vi "TR_Load_TDMS_for_Repair.vi"(6 "Basic setings cluster":variant, 7 "Decimate?":bool, 8 "error in (no error)":errorcluster, 9 "Post-processing parameters in":variant, 10 "Full settings cluster":variant, 11 "TDMS track":path) -> (0 "error out":errorcluster, 2 "Post-processing parameters out (copy)":variant, 3 "XY data":T1)   [LabVIEW 2018, in "Tracks Repair.lvlib"]
uses:
  Tracks Repair.lvlib
  SubVi's/Controls/CTL_Overlays_cluster.ctl
  SubVi's/Controls/CTL_Full_Track_Array.ctl
  <vilib>/Utility/miscctls.llb/LVBoundsTypeDef.ctl
  SubVi's/Controls/CTL_Settings_cluster.ctl
  SubVi's/Controls/CTL_Histogram_parameters.ctl
  SubVi's/Controls/CTL_Filter_selector.ctl
  SubVi's/Controls/CTL_Acquisition_speed_selector.ctl
  SubVi's/Controls/CTL_Segmented_plot_parameters.ctl
  SubVi's/Controls/CTL_IO_params_cluster.ctl
  SubVi's/Controls/CTL_Conditions_Array.ctl
  SubVi's/Controls/CTL_Conditions_Cluster.ctl
  SubVi's/Controls/CTL_Condition_type.ctl
  SubVi's/Controls/CTL_Comparison_type.ctl
  SubVi's/Controls/CTL_Validity_check_criteria.ctl
  SubVi's/Controls/CTL_Response_info.ctl
  SubVi's/Controls/CTL_Condition_response_type.ctl
  SubVi's/Controls/CTL_Reponse_port_info.ctl
  SubVi's/Controls/CTL_Calibration_parameters.ctl
  SubVi's/Controls/CTL_Dispenser_calibration_info.ctl
  SubVi's/Controls/CTL_Post-processing_params.ctl
  SubVi's/Controls/CTL_Mouse_Draw_Params.ctl
  <vilib>/vision/Image Controls.llb/IMAQ Image.ctl
  SubVi's/Controls/CTL_Pixel_to_Zone_array.ctl
  SubVi's/Controls/CTL_Basic_cage_settings.ctl
  Tracker.lvlib
  Common_Resources.lvlib
panel:
  out "Overlays cluster out":T2
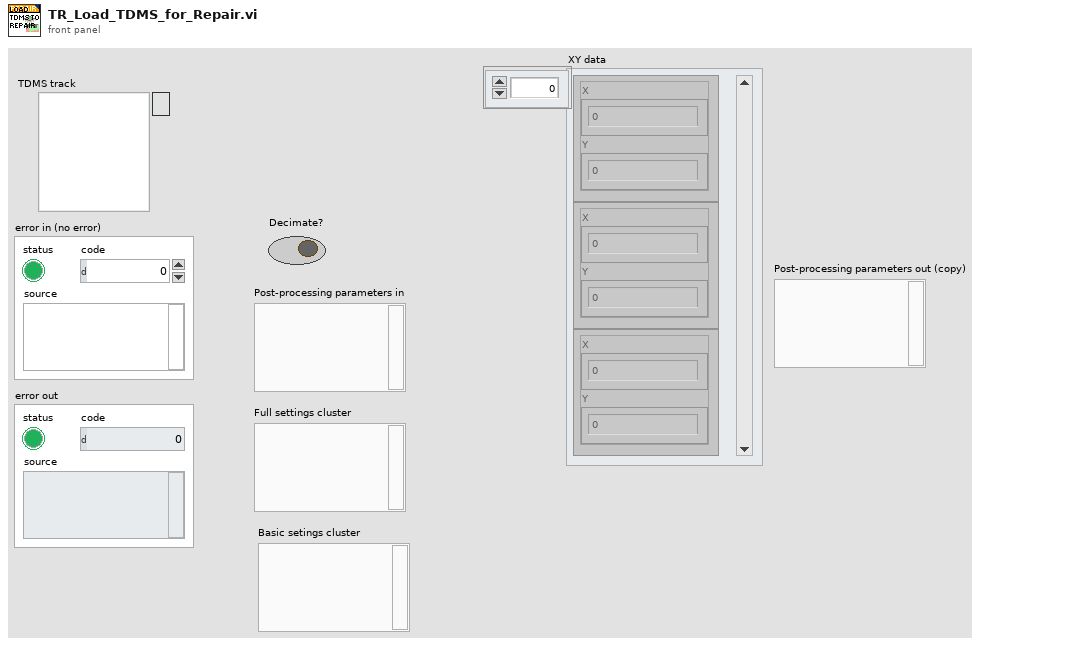
[diagram p1: front panel]
types:
  T1 = typedef "Common_Resources.lvlib/CTL_Full_Track_Array.ctl" = cluster{"X":dbl, "Y":dbl}[]
  T2 = typedef "Common_Resources.lvlib/CTL_Overlays_cluster.ctl" = cluster{"Time-coded track overlay (array)":u32[][], "Speed-coded track overlay (array)":u32[][], "Plain track overlay pixmap":u32[][], "Location density map image":u32[][], "Speed density map image":u32[][], "Location density map":dbl[][], "Speed density map":dbl[][]}
  T3 = typedef "Common_Resources.lvlib/CTL_Basic_cage_settings.ctl" = cluster{"Vert. offset":dbl, "Hor. offset":dbl, "Bridge swap":bool, "Twisted neck":bool, "Cage diam.":i32, "Magn.rot.":i32, "Acq. speed":dbl}
  T4 = typedef "Common_Resources.lvlib/CTL_Post-processing_params.ctl" = cluster{"Defragment TDMS? (F)":bool, "Start time (SW)":timestamp, "Start time (HW)":u32, "Data filtering":T5, "Mouse drawing parameters":T6, "Size of the image (480x480)":cluster{"X size":dbl, "Y size":dbl}, "Image ref. in":T7, "Calibration parameters":T8, "Pixel to zone":T10}
  T5 = typedef "Common_Resources.lvlib/CTL_Filter_selector.ctl" = cluster{"Filter type":enum16{"None", "Savitzky-Golay"}, "Length":i32, "Order":i32}
  T6 = typedef "Common_Resources.lvlib/CTL_Mouse_Draw_Params.ctl" = cluster{"Trace length, samples":u16, "Rainbow track":bool, "Rainbow track is speed":bool, "Bright mouse lineout":bool, "Colors array":u32[], "Pixels per mm":dbl}
  T7 = typedef "IMAQ Image.ctl" = refnum<image>
  T8 = typedef "Common_Resources.lvlib/CTL_Calibration_parameters.ctl" = cluster{"Timing calibration sw/hw":dbl, "True FPS":dbl, "True frame time, s":dbl, "Disp. calibration info":T9}
  T9 = typedef "Common_Resources.lvlib/CTL_Dispenser_calibration_info.ctl" = cluster{"Channel":u8, "Speed, µl per ms":dbl}[]
  T10 = typedef "Common_Resources.lvlib/CTL_Pixel_to_Zone_array.ctl" = i8[][]
  T11 = typedef "Common_Resources.lvlib/CTL_Settings_cluster.ctl" = cluster{"Defaults":cluster{"Default User":dbl, "VISA Resource Name ":string, "Histogram parameters":T12}, "Recording and saving":cluster{"Researcher name":string, "Name prefix":string, "Data post-processing":T5, "Stop at":dbl, "\"Stop at\" enabled":bool, "Default save folder path":path, "Acquisition FPS":T13}, "Geometry":T14, "IO parameters":T15, "Conditions presets array":T16, "Calibration parameters":T8, "Settings loaded OK":bool}
  T12 = typedef "Common_Resources.lvlib/CTL_Histogram_parameters.ctl" = cluster{"max":dbl, "min":dbl, "# bins":i32, "threshold":dbl, "thr. type":enum16{"higher accepted", "lower accepted"}}
  T13 = typedef "Common_Resources.lvlib/CTL_Acquisition_speed_selector.ctl" = enum16{"Max", "Optimal", "Eco"}
  T14 = typedef "Common_Resources.lvlib/CTL_Segmented_plot_parameters.ctl" = cluster{"Cage diameter, mm":u16, "Starting angle MIDFIELD":i16, "Starting angle BORDER":i16, "Radius, mm CENTER":u16, "Radius, mm MIDFIELD":u16, "N segments MIDFIELD":u8, "N segments BORDER":u8, "R-gap, mm":sgl, "Bridge swap":bool, "Bridge H. offset":sgl, "Bridge V. offset":sgl, "Twisted neck":bool, "Alt. magn. orientation":bool, "Sensor board size":enum16{"Small", "Large"}}
  T15 = typedef "Common_Resources.lvlib/CTL_IO_params_cluster.ctl" = cluster{"IO general config.":u16, "IO 1 configuration":u16, "IO 2 configuration":u16, "IO 3 configuration":u16, "IO 4 configuration":u16, "Activate ext. RS-232":u16, "IO inversion config.":u16, "Sync capability":u8}
  T16 = typedef "Common_Resources.lvlib/CTL_Conditions_Array.ctl" = T17[]
  T17 = typedef "Common_Resources.lvlib/CTL_Conditions_Cluster.ctl" = cluster{"Enabled":bool, "Name":string, "Specifier(s)":cluster{"Specifier enabled":bool, "Condition type":T18, "Comparison type":T19, "Value":dbl, "Validity criteria(s)":cluster{"V. check enabled":bool, "Criteria":T20, "Validity value":dbl}[]}[], "Response":T21, "Has been set":bool}
  T18 = typedef "Common_Resources.lvlib/CTL_Condition_type.ctl" = enum16{"Speed", "Zone", "Angle to wall"}
  T19 = typedef "Common_Resources.lvlib/CTL_Comparison_type.ctl" = enum16{"Less", "Less or Equal", "Equal", "Greater or Equal", "Greater", "Not Equal"}
  T20 = typedef "Common_Resources.lvlib/CTL_Validity_check_criteria.ctl" = enum16{"Running bout (seconds)", "Running bout (meters)"}
  T21 = typedef "Common_Resources.lvlib/CTL_Response_info.ctl" = cluster{"Response type":T22, "TTL port":T23, "TTL pulse length, ms":dbl}
  T22 = typedef "Common_Resources.lvlib/CTL_Condition_response_type.ctl" = enum16{"None", "Air puff", "Liquid reward"}
  T23 = typedef "Common_Resources.lvlib/CTL_Reponse_port_info.ctl" = enum16{"Port 1", "Port 2", "Port 3", "Port 4"}
  T24 = typedef "LVBoundsTypeDef.ctl" = cluster{"Width":u32, "Height":u32}
  T25 = typedef "Common_Resources.lvlib/CTL_Cage_Coords_(arrays).ctl" = cluster{"R from center":dbl[], "sin(a)":dbl[], "Mouse Xc":dbl[], "Mouse Yc":dbl[], "X1-X2":dbl[], "Y1-Y2":dbl[], "Cage Xc":dbl[], "Cage Yc":dbl[], "Frame time, s":dbl}
  T26 = typedef "Common_Resources.lvlib/CTL_Animal_Coordinates_and_Speed_(arr).ctl" = cluster{"R from center":dbl[], "phi (mouse angular position in the cage)":dbl[], "alpha (mouse rot. angle)":dbl[], "X":dbl[], "Y":dbl[], "theta (from center towards mouse)":dbl[], "beta (cage rot. against mouse)":dbl[], "w (mouse angle to wall)":dbl[], "Speed (filtered)":dbl[], "Zone":i8[]}
  T27 = cluster{"Boolean Round":bool, "code":i32, "source":string}
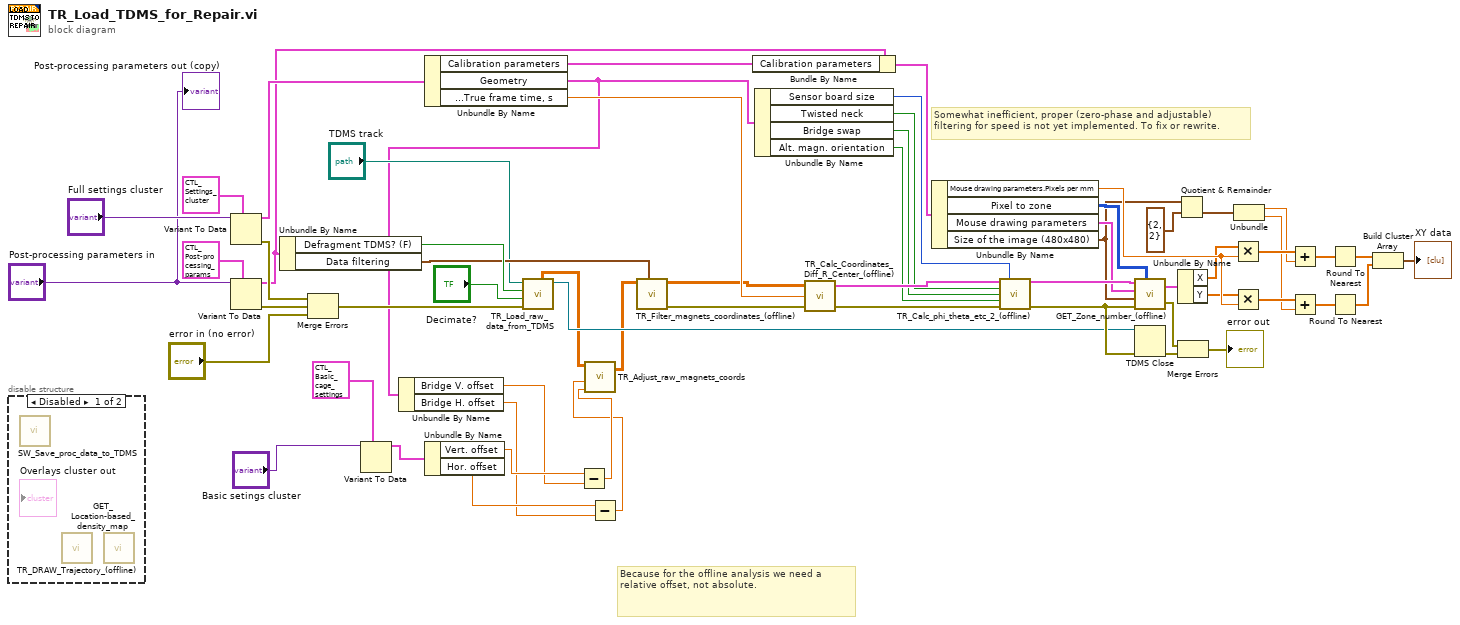
[diagram p0: block diagram]
diagram:
  # "Because for the offline analysis we need a relative offset, not absolute."
  # "Somewhat inefficient, proper (zero-phase and adjustable) filtering for speed is not yet implemented. To fix or rewrite."
  n1 = disable-structure shown="Disabled" {
    frame Disabled {
      n2 = call "SW_Save_proc_data_to_TDMS.vi"() -> ()  [unwired: 11 in, 1 out]
      n3 = call "TR_DRAW_Trajectory_(offline).vi"() -> ()  [unwired: 13 in, 3 out]
      n4 = call "GET_Location-based_density_map.vi"() -> ()  [unwired: 13 in, 3 out]
    }
    frame Enabled {
    }
  }
  n5 = Variant To Data(type=T11 {"Defaults"={"Default User"=0.0, "VISA Resource Name "="", "Histogram parameters"={"max"=300.0, "min"=0.0, "# bins"=10, "threshold"=8.0, "thr. type"=enum."higher accepted"}}, "Recording and saving"={"Researcher name"="", "Name prefix"="", "Data post-processing"={"Filter type"=enum."None", "Length"=0, "Order"=0}, "Stop at"=0.0, "\"Stop at\" enabled"=FALSE, "Default save folder path"=path "", "Acquisition FPS"=enum."Max"}, "Geometry"={"Cage diameter, mm"=0, "Starting angle MIDFIELD"=0, "Starting angle BORDER"=0, "Radius, mm CENTER"=0, "Radius, mm MIDFIELD"=0, "N segments MIDFIELD"=0, "N segments BORDER"=0, "R-gap, mm"=0.0, "Bridge swap"=FALSE, "Bridge H. offset"=0.0, "Bridge V. offset"=0.0, "Twisted neck"=FALSE, "Alt. magn. orientation"=FALSE, "Sensor board size"=enum."Small"}, "IO parameters"={"IO general config."=0, "IO 1 configuration"=0, "IO 2 configuration"=0, "IO 3 configuration"=0, "IO 4 configuration"=0, "Activate ext. RS-232"=0, "IO inversion config."=0, "Sync capability"=0}, "Conditions presets array"=[], "Calibration parameters"={"Timing calibration sw/hw"=0.0, "True FPS"=0.0, "True frame time, s"=0.0, "Disp. calibration info"=[]}, "Settings loaded OK"=FALSE} ("Settings cluster"), Variant="Full settings cluster") -> (data=w20:T11, error out=w18:errorcluster)  [unwired: 1 in]
  n6 = Variant To Data(type=T4 {"Defragment TDMS? (F)"=FALSE, "Start time (SW)"=timestamp(0 s since 1904-01-01), "Start time (HW)"=0, "Data filtering"={"Filter type"=enum."Savitzky-Golay", "Length"=41, "Order"=3}, "Mouse drawing parameters"={"Trace length, samples"=0, "Rainbow track"=FALSE, "Rainbow track is speed"=FALSE, "Bright mouse lineout"=FALSE, "Colors array"=[], "Pixels per mm"=0.0}, "Size of the image (480x480)"={"X size"=480.0, "Y size"=480.0}, "Image ref. in"=refnum, "Calibration parameters"={"Timing calibration sw/hw"=1.0, "True FPS"=80.0, "True frame time, s"=0.0125, "Disp. calibration info"=[]}, "Pixel to zone"=[]} ("Processing parameters"), Variant="Post-processing parameters in") -> (data=w17:T4, error out=w16:errorcluster)  [unwired: 1 in]
  n7 = Unbundle By Name(w17) -> ("Defragment TDMS? (F)"=w53:bool, "Data filtering"=w52:T5)
  n8 = Merge Errors(w18, w16, "error in (no error)") -> (w19:errorcluster)
  n9 = Variant To Data(type=T3 {"Vert. offset"=48.0, "Hor. offset"=0.0, "Bridge swap"=FALSE, "Twisted neck"=FALSE, "Cage diam."=325, "Magn.rot."=0, "Acq. speed"=100.01280589338842} ("Settings"), Variant="Basic setings cluster") -> (data=w8:T3)  [unwired: 1 in, 1 out]
  n10 = Unbundle By Name(w20) -> ("Calibration parameters"=w51:T8, "Geometry"=w7:T14, "Calibration parameters.True frame time, s"=w60:dbl)
  n11 = Unbundle By Name(w7) -> ("Bridge V. offset"=w5:sgl, "Bridge H. offset"=w3:sgl)
  n12 = Unbundle By Name(w8) -> ("Vert. offset"=w6:dbl, "Hor. offset"=w4:dbl)
  n13 = call "TR_Load_raw_data_from_TDMS.vi"("error in (no error)"=w19, "Decimate?"="Decimate?", "Defragment TDMS? (F)"=w53, "TDMS track ref. in"="TDMS track") -> ("TDMS track ref. out"=w41:refnum<k34>, "Raw values"=w13:dbl[][])  [unwired: 2 in, 4 out]
  n14 = Subtract(x=w6, y=w5) -> (x-y=w2:dbl)
  n15 = Subtract(x=w4, y=w3) -> (x-y=w1:dbl)
  n16 = call "TR_Adjust_raw_magnets_coords.vi"("Offset V."=w2, "Offset H."=w1, "Raw values in"=w13) -> ("Off-values out"=w12:dbl[][])  [unwired: 4 in]
  n17 = call "TR_Filter_magnets_coordinates_(offline).vi"("Data filtering"=w52, "Magnets raw coordinates in"=w12) -> ("error out"=w61:errorcluster, "Magnets filtered coordinates out"=w59:dbl[][])  [unwired: 8 in]
  n18 = Bundle By Name(cluster=w17, "Calibration parameters"=w51) -> (w50:T4)
  n19 = Unbundle By Name(w7) -> ("Sensor board size"=w54:enum16{"Small", "Large"}, "Twisted neck"=w56:bool, "Bridge swap"=w55:bool, "Alt. magn. orientation"=w11:bool)
  n20 = call "TR_Calc_Coordinates_Diff_R_Center_(offline).vi"("Error In"=w61, "Frame time, s"=w60, "Magnets coordinates in"=w59) -> ("Error Out"=w58:errorcluster, "Output cluster of data"=w57:T25)  [unwired: 1 in]
  n21 = Unbundle By Name(w50) -> ("Mouse drawing parameters.Pixels per mm"=w46:dbl, "Pixel to zone"=w47:T10, "Mouse drawing parameters"=w48:T6, "Size of the image (480x480)"=w45:cluster{"X size":dbl, "Y size":dbl})
  n22 = call "TR_Calc_phi_theta_etc_2_(offline).vi"("Input data cluster"=w57, "SB size"=w54, "Twisted neck"=w56, "Bridge swap"=w55, "Use alternative magnets orientation"=w11, "Error In"=w58) -> ("Animal coordinates cluster"=w49:T26, "Error out"=w42:errorcluster)  [unwired: 8 in]
  n23 = call "GET_Zone_number_(offline).vi"("Animal coordinates cluster in"=w49, "Mouse drawing parameters"=w48, "Size of the image (480x480)"=w45, "error in (no error)"=w42, "Array of the pixel to zone correspondences"=w47) -> ("Animal coordinates cluster out"=w39:T26, "error out"=w25:T27)
  n24 = TDMS Close(8:w42, 11:w41) -> (0:w26:errorcluster)  [unwired: 1 out]
  n25 = Quotient & Remainder(x=w45, y=T24 {"Width"=2, "Height"=2}) -> (floor(x/y)=w29:cluster{dbl, dbl})  [unwired: 1 out]
  n26 = Unbundle By Name(w39) -> ("X"=w33:dbl[], "Y"=w31:dbl[])
  n27 = Merge Errors(w25, w26) -> (→"error out":errorcluster)
  n28 = Multiply(x=w33, y=w46) -> (x*y=w32:dbl[])
  n29 = Multiply(x=w31, y=w46) -> (x*y=w36:dbl[])
  n30 = Unbundle(w29) -> (w28:dbl, w27:dbl)
  n31 = Add(x=w32, y=w28) -> (x+y=w38:dbl[])
  n32 = Add(x=w36, y=w27) -> (x+y=w35:dbl[])
  n33 = Round To Nearest(number=w38) -> (nearest integer value=w37:dbl[])
  n34 = Round To Nearest(number=w35) -> (nearest integer value=w34:dbl[])
  n35 = Build Cluster Array(w37, w34) -> (→"XY data":cluster{dbl, dbl}[])
  "Post-processing parameters out (copy)" <- "Post-processing parameters in"
